vi "MessageQueue_RemoveEntryByNameQueue.vi"(0 "Queue in":refnum<queue>, 2 "CommandName":string, 5 "error in (no error)":errorcluster) -> (14 "Queue out":refnum<queue>, 19 "error out":errorcluster)   [LabVIEW 2016]
doc: "Löscht Queueelemente mit dem CommandName aus einer Queue heraus"
uses:
  private/MessageQueue.MessageTypeDef.ctl
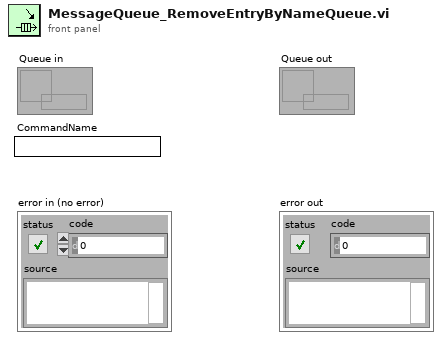
[diagram p1: front panel]
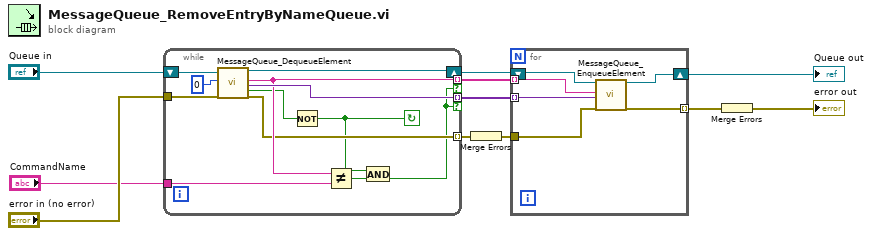
[diagram p0: block diagram]
diagram:
  n1 = while {
    tunnel: [w21] -> w5 mode=indexing if=w13
    tunnel: [w20] -> w4 mode=indexing if=w13
    shift-right: [w18] -> w6
    shift-left: "Queue in" -> [w23]
    tunnel: "error in (no error)" -> [w17]
    tunnel: [w16] -> w9 mode=indexing
    tunnel: "CommandName" -> [w15]
    stop <- w12 continue-if-true
    n2 = call "MessageQueue_DequeueElement.vi"("QueueIn"=w23, "Timeout"=0, "ErrorIn"=w17) -> ("QueueOut"=w18:refnum<queue>, "Message"=w20:string, "Data"=w21:variant, "Timeout"=w14:bool, "ErrorOut"=w16:errorcluster)  [unwired: 12 in]
    n3 = Not(x=w14) -> (.not. x?=w12:bool)
    n4 = Not Equal?(x=w20, y=w15) -> (x != y?=w19:bool)
    n5 = And(x=w12, y=w19) -> (x .and. y?=w13:bool)
  }
  n6 = Merge Errors(w9) -> (w10:errorcluster)
  n7 = for {
    tunnel: w4 -> [w29] mode=indexing
    tunnel: w5 -> [w28] mode=indexing
    shift-right: [w26] -> w11
    shift-left: w6 -> [w27]
    tunnel: [w25] -> w7 mode=indexing
    tunnel: w10 -> [w24]
    n8 = call "MessageQueue_EnqueueElement.vi"("QueueIn"=w27, "Message"=w29, "Data"=w28, "ErrorIn"=w24) -> ("QueueOut"=w26:refnum<queue>, "ErrorOut"=w25:errorcluster)  [unwired: 14 in]
  }
  "Queue out" <- w11
  n9 = Merge Errors(w7) -> (→"error out":errorcluster)
